vi "Single Shot Pulse Sequence - 2nd Setup.vi"() -> ()   [LabVIEW 2024]
uses:
  <instrlib>/niFgen/niFgen.llb/niFgen Waveform Type.ctl
  <instrlib>/niFgen/niFgen.llb/niFgen_ctl Trigger DigEdge - Edge Values (Ring).ctl
  <instrlib>/niFgen/niFgen.llb/niFgen_ctl Trigger Source Values (Ring).ctl
  <instrlib>/niFgen/niFgen.llb/niFgen Trigger Mode.ctl
  <instrlib>/niScope/Controls/niScope acquisition type.ctl
  <instrlib>/niScope/Controls/niScope trigger slope.ctl
  <instrlib>/niScope/Controls/niScope trigger source.ctl
  <instrlib>/niFgen/niFgen.llb/niFgen Output Mode.ctl
  <instrlib>/niScope/Configure/Trigger/niScope Configure Trigger Edge.vi
  <vilib>/Utility/file.llb/Read Delimited Spreadsheet (DBL).vi
  <instrlib>/niFgen/niFgen.llb/niFgen Create Waveform (DBL).vi
  <instrlib>/niFgen/niFgen.llb/niFgen Configure Digital Edge Start Trigger.vi
  <instrlib>/niScope/Acquire/Fetch/niScope Fetch Cluster.vi
  <vilib>/Waveform/WDTFileIO.llb/Export Waveform To Spreadsheet File.vi
panel:
  in  "Boolean":bool
  in  "HP Amplifier":enum16{"PE15A4017", "ZHL-1-2W-S+", "ZHL-5W-1X+"}(ring)=enum."ZHL-1-2W-S+"
  in  "Larmor Frequency":dbl=27320000.0 caption="Frequency" format="%.4p"
  in  "Pulse Train File":path=path "C:/Users/MK92/OneDrive - University of South Carolina/Github Repos/Compact-NMR/System_development/Van-Hove/LabVIEW/7 us 90 Degree - 1.25 ms Tau - 4 Pulses.txt"
  out "Pulse Echo":waveform(dbl)(graph)={"t0"=timestamp(0 s since 1904-01-01), "dt"=3.3333333333333333e-06, "Y"=array[1500 elements]} caption="Waveform Graph"
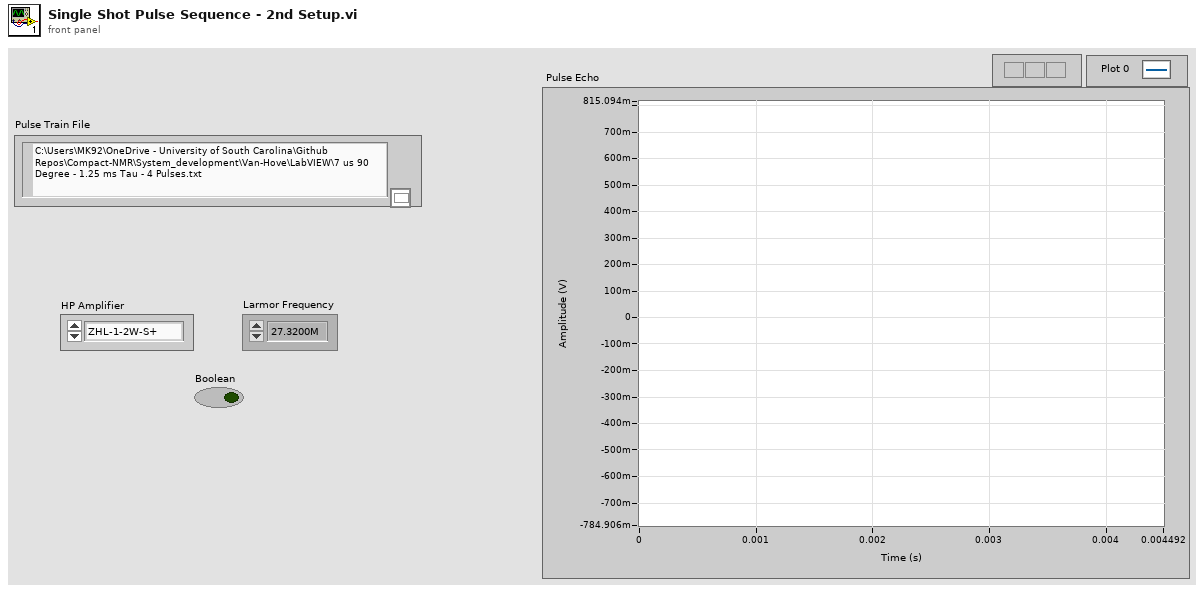
[diagram p1: front panel]
types:
  T1 = typedef "niFgen Output Mode.ctl" = u32
  T2 = typedef "niScope trigger source.ctl" = string
  T3 = typedef "niScope trigger slope.ctl" = i32
  T4 = typedef "niScope acquisition type.ctl" = i32
  T5 = typedef "niFgen Trigger Mode.ctl" = i32
  T6 = typedef "niFgen_ctl Trigger Source Values (Ring).ctl" = string
  T7 = typedef "niFgen_ctl Trigger DigEdge - Edge Values (Ring).ctl" = i32
  T8 = typedef "niFgen Waveform Type.ctl" = i32
  T9 = cluster{"relativeInitialX":dbl, "xIncrement":dbl, "wfm":dbl[]}
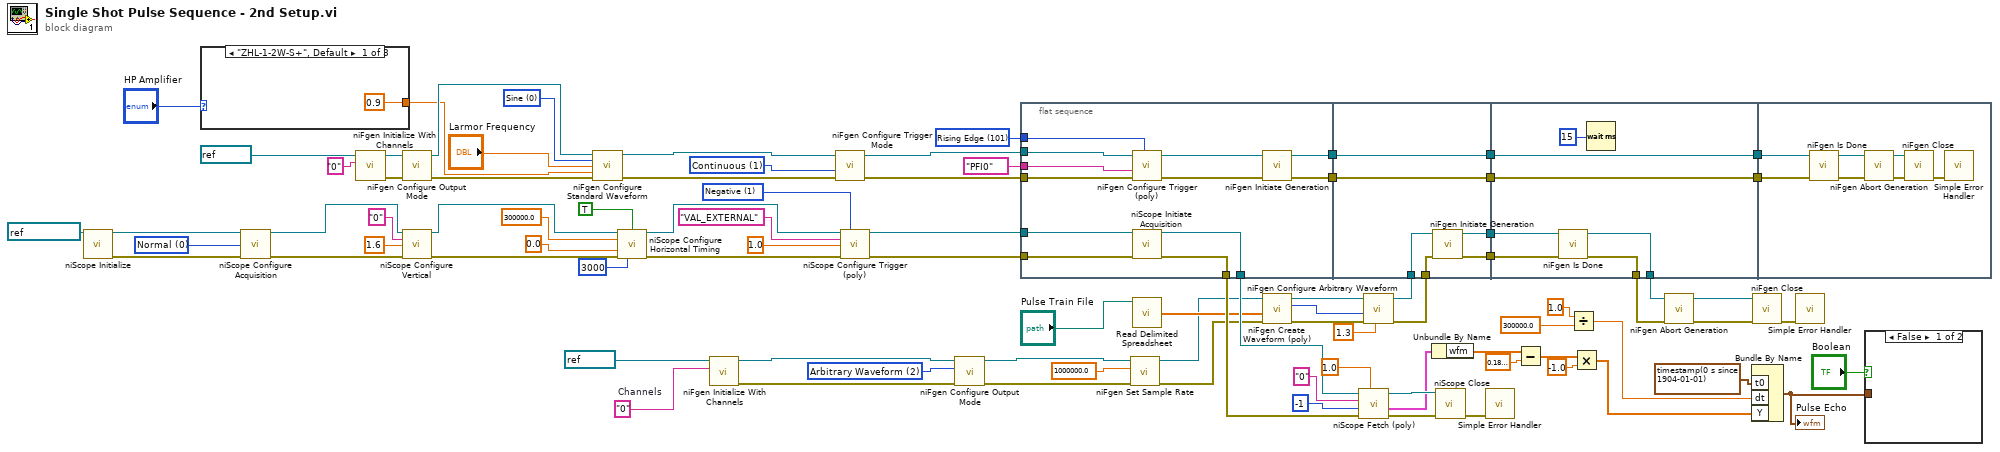
[diagram p0: block diagram]
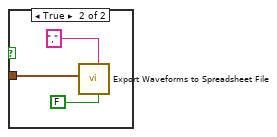
[diagram p2: hidden frame]
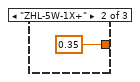
[diagram p3: hidden frame]
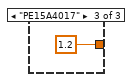
[diagram p4: hidden frame]
diagram:
  w16 = "0"  # Channels
  w15 = T1 2 items=["Standard Function", "Frequency List", "Arbitrary Waveform", "Arbitrary Sequence", "Script"] ("output mode")
  w55 = T3 1 items=["Positive", "Negative"] ("trigger slope")
  w56 = T4 0 items=["Normal"=0, "Flex Res"=1, "DDC"=3] ("acquisition Type")
  w68 = T5 1 items=["Single", "Continuous", "Stepped", "Burst"] ("Trigger Mode (default: 1=continuous)")
  w72 = T7 101 items=["Rising Edge"=101, "Falling Edge"=102] ("Edge (Rising)")
  w73 = T8 0 items=["Sine", "Square", "Triangle", "Ramp Up", "Ramp Down", "DC", "Noise", "User"] ("Waveform")
  n1 = call <instrlib>:"niScope Initialize.vi"("resource name"=refnum<k15> "PXI1Slot4") -> ("instrument handle"=w57:refnum<k15>, "error out"=w58:errorcluster)  [unwired: 13 in]
  n2 = case shown="\"ZHL-1-2W-S+\", Default" "HP Amplifier" {
    tunnel: [0.9 ("Amplitude") 0.35 ("Amplitude") 1.2 ("Amplitude")] -> w3
    frame "ZHL-1-2W-S+", Default {
    }
    frame "ZHL-5W-1X+" {
    }
    frame "PE15A4017" {
    }
  }
  n3 = call <instrlib>:"niScope Configure Acquisition.vi"("instrument handle"=w57, "acquisition Type"=w56, "error in"=w58) -> ("instrument handle out"=w59:refnum<k15>, "error out"=w60:errorcluster)  [unwired: 11 in]
  n4 = call <instrlib>:"niFgen Initialize With Channels.vi"("Channel Name"="0", "Resource Name"=refnum<k15> "Dev2" ("Sine Wave Module")) -> ("error out"=w78:errorcluster, "Instrument Handle Out"=w81:refnum<k15>)  [unwired: 8 in]
  n5 = call <instrlib>:"niFgen Configure Output Mode.vi"("error in (no error)"=w78, "Instrument Handle"=w81) -> ("error out"=w77:errorcluster, "Instrument Handle Out"=w80:refnum<k15>)  [unwired: 7 in]
  n6 = call <instrlib>:"niScope Configure Vertical.vi"("instrument handle"=w59, "channels"="0", "vertical range"=1.6, "error in"=w60) -> ("instrument handle out"=w61:refnum<k15>, "error out"=w62:errorcluster)  [unwired: 10 in]
  n7 = call <instrlib>:"niFgen Configure Standard Waveform.vi"("Instrument Handle"=w80, "Waveform"=w73, "Frequency"="Larmor Frequency", "Amplitude"=w3, "error in (no error)"=w77) -> ("Instrument Handle Out"=w79:refnum<k15>, "error out"=w76:errorcluster)  [unwired: 9 in]
  n8 = call <instrlib>:"niScope Configure Horizontal Timing.vi"("instrument handle"=w61, "enforce realtime"=TRUE, "min sample rate"=300000.0, "reference position"=0.0, "error in"=w62, "min record length"=3000) -> ("instrument handle out"=w63:refnum<k15>, "error out"=w64:errorcluster)  [unwired: 8 in]
  n9 = call <instrlib>:"niFgen Initialize With Channels.vi"("Channel Name"=w16, "Resource Name"=refnum<k15> "Dev1" ("FGEN Resource Name 2")) -> ("error out"=w19:errorcluster, "Instrument Handle Out"=w20:refnum<k15>)  [unwired: 8 in]
  n10 = call <instrlib>:"niFgen Configure Trigger Mode.vi"("error in (no error)"=w76, "Trigger Mode (default: 1=continuous)"=w68, "Instrument Handle"=w79) -> ("error out"=w71:errorcluster, "Instrument Handle Out"=w69:refnum<k15>)  [unwired: 7 in]
  n11 = call-poly <instrlib>:"niScope Configure Trigger (poly).vi"("instrument handle"=w63, "trigger slope"=w55, "trigger source"=T2 "VAL_EXTERNAL", "trigger level"=1.0, "error in"=w64) -> ("instrument handle out"=w49:refnum<k15>, "error out"=w48:errorcluster)  [unwired: 9 in]
  n12 = call <instrlib>:"niFgen Configure Output Mode.vi"("error in (no error)"=w19, "Output Mode (default: 0=Standard Function)"=w15, "Instrument Handle"=w20) -> ("error out"=w23:errorcluster, "Instrument Handle Out"=w22:refnum<k15>)  [unwired: 6 in]
  n13 = flat-sequence {
    tunnel: w49 -> [w98]
    tunnel: w48 -> [w97]
    tunnel: [w96] -> w47
    tunnel: [w95] -> w46
    tunnel: [w94] -> w89
    tunnel: [w93] -> w88
    tunnel: w72 -> [w103]
    tunnel: w71 -> [w102]
    tunnel: T6 "PFI0" ("Source") -> [w101]
    tunnel: w69 -> [w100]
    tunnel: w14 -> [w110]
    tunnel: w13 -> [w109]
    tunnel: [w108] -> w87
    tunnel: [w107] -> w86
    tunnel: [w106] -> w85
    tunnel: w89 -> [w106]
    tunnel: [w105] -> w84
    tunnel: w88 -> [w105]
    tunnel: [w116] -> w67
    tunnel: [w115] -> w66
    tunnel: w87 -> [w114]
    tunnel: w86 -> [w113]
    tunnel: [w112] -> w83
    tunnel: w85 -> [w112]
    tunnel: [w111] -> w82
    tunnel: w84 -> [w111]
    tunnel: w83 -> [w119]
    tunnel: w82 -> [w118]
    frame #0 {
      n14 = call-poly <instrlib>:"niFgen Configure Trigger (poly).vi"("Edge (Rising)"=w103, "error in (no error)"=w102, "Source"=w101, "Instrument Handle"=w100) -> ("error out"=w99:errorcluster, "Instrument Handle Out"=w104:refnum<k15>)  [unwired: 6 in]
      n15 = call <instrlib>:"niScope Initiate Acquisition.vi"("instrument handle"=w98, "error in"=w97) -> ("instrument handle out"=w96:refnum<k15>, "error out"=w95:errorcluster)  [unwired: 12 in]
      n16 = call <instrlib>:"niFgen Initiate Generation.vi"("error in (no error)"=w99, "Instrument Handle"=w104) -> ("error out"=w93:errorcluster, "Instrument Handle Out"=w94:refnum<k15>)  [unwired: 8 in]
    }
    frame #1 {
      n17 = call <instrlib>:"niFgen Initiate Generation.vi"("error in (no error)"=w110, "Instrument Handle"=w109) -> ("error out"=w107:errorcluster, "Instrument Handle Out"=w108:refnum<k15>)  [unwired: 8 in]
    }
    frame #2 {
      n18 = call <instrlib>:"niFgen Is Done.vi"("error in (no error)"=w113, "Instrument Handle"=w114) -> ("error out"=w116:errorcluster, "Instrument Handle Out"=w115:refnum<k15>)  [unwired: 7 in, 1 out]
      n19 = Wait (ms)(milliseconds to wait=u32 15) -> ()  [unwired: 1 out]
    }
    frame #3 {
      n20 = call <instrlib>:"niFgen Is Done.vi"("error in (no error)"=w118, "Instrument Handle"=w119) -> ("error out"=w122:errorcluster, "Instrument Handle Out"=w121:refnum<k15>)  [unwired: 7 in, 1 out]
      n21 = call <instrlib>:"niFgen Abort Generation.vi"("error in (no error)"=w122, "Instrument Handle"=w121) -> ("error out"=w123:errorcluster, "Instrument Handle Out"=w124:refnum<k15>)  [unwired: 8 in]
      n22 = call <instrlib>:"niFgen Close.vi"("error in (no error)"=w123, "Instrument Handle"=w124) -> ("error out"=w120:errorcluster)  [unwired: 9 in]
      n23 = call <vilib>:"Simple Error Handler.vi"("error in (no error)"=w120) -> ()  [unwired: 4 in, 5 out]
    }
  }
  n24 = call <instrlib>:"niFgen Set Sample Rate.vi"("error in (no error)"=w23, "Sample Rate (Samp/s)"=1000000.0 ("Sample Rate"), "Instrument Handle"=w22) -> ("error out"=w26:errorcluster, "Instrument Handle Out"=w25:refnum<k15>)  [unwired: 7 in]
  n25 = call-poly <vilib>:"Read Delimited Spreadsheet.vi"("file path (dialog if empty)"="Pulse Train File") -> ("first row"=w27:dbl[])  [unwired: 9 in, 5 out]
  n26 = call-poly <instrlib>:"niFgen Create Waveform (poly).vi"("error in (no error)"=w26, "Waveform Data Array"=w27, "Instrument Handle"=w25) -> ("error out"=w29:errorcluster, "Waveform Handle"=w30:i32, "Instrument Handle Out"=w28:refnum<k15>)  [unwired: 6 in]
  n27 = call-poly <instrlib>:"niScope Fetch (poly).vi"("timeout"=1.0, "error in"=w46, "numSamples"=-1, "channels"="0", "instrument handle"=w47) -> ("error out"=w39:errorcluster, "waveform"=w37:T9, "instrument handle out"=w40:refnum<k15>)  [unwired: 3 in, 1 out]
  n28 = call <instrlib>:"niFgen Configure Arbitrary Waveform.vi"("Gain"=1.3, "error in (no error)"=w29, "Waveform Handle"=w30, "Instrument Handle"=w28) -> ("error out"=w14:errorcluster, "Instrument Handle Out"=w13:refnum<k15>)  [unwired: 6 in]
  n29 = Unbundle By Name(w37) -> ("wfm"=w32:dbl[])
  n30 = call <instrlib>:"niScope Close.vi"("instrument handle"=w40, "error in"=w39) -> ("error out"=w65:errorcluster)  [unwired: 13 in]
  n31 = call <vilib>:"Simple Error Handler.vi"("error in (no error)"=w65) -> ()  [unwired: 4 in, 5 out]
  n32 = Subtract(x=w32, y=0.18000000000000002) -> (x-y=w7:dbl[])
  n33 = Divide(x=1.0, y=300000.0) -> (x/y=w36:dbl)
  n34 = Multiply(x=w7, y=-1.0) -> (x*y=w6:dbl[])
  n35 = call <instrlib>:"niFgen Abort Generation.vi"("error in (no error)"=w67, "Instrument Handle"=w66) -> ("error out"=w8:errorcluster, "Instrument Handle Out"=w9:refnum<k15>)  [unwired: 8 in]
  n36 = Bundle By Name("t0"=timestamp(0 s since 1904-01-01), "dt"=w36, "Y"=w6) -> (w2:waveform(dbl))  [unwired: 1 in]
  "Pulse Echo" <- w2
  n37 = call <instrlib>:"niFgen Close.vi"("error in (no error)"=w8, "Instrument Handle"=w9) -> ("error out"=w10:errorcluster)  [unwired: 9 in]
  n38 = call <vilib>:"Simple Error Handler.vi"("error in (no error)"=w10) -> ()  [unwired: 4 in, 5 out]
  n39 = case shown="False" "Boolean" {
    tunnel: w2 -> [_ w125]
    frame False {
    }
    frame True {
      n40 = call-poly <vilib>:"Export Waveforms to Spreadsheet File.vi"("header? (write header:T)"=FALSE, "delimiter (Tab)"=",", "waveform"=w125) -> ()  [unwired: 7 in, 2 out]
    }
  }
